vi "0 to 99 sub vi.vi"(1 "Numeric":dbl) -> (0 "String":string)   [LabVIEW 2020]
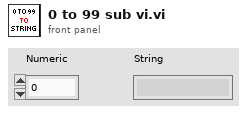
[diagram p1: front panel]
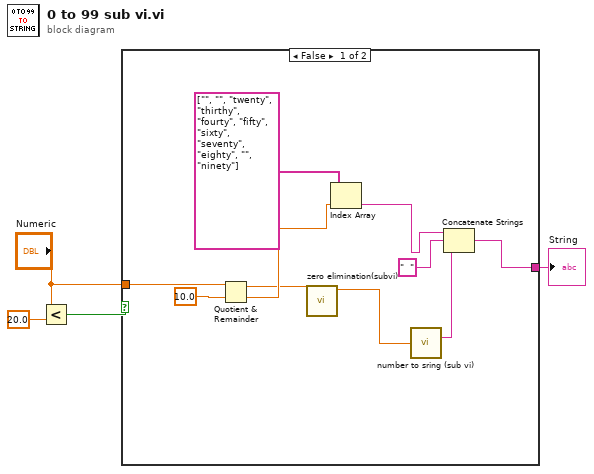
[diagram p0: block diagram]
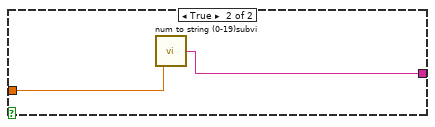
[diagram p2: hidden frame]
diagram:
  n1 = Less?(x="Numeric", y=20.0) -> (x < y?=w1:bool)
  n2 = case shown="False" w1 {
    tunnel: "Numeric" -> [w14 w16]
    tunnel: [w9 w15] -> w4
    frame False {
      n3 = Quotient & Remainder(x=w14, y=10.0) -> (x-y*floor(x/y)=w7:dbl, floor(x/y)=w8:dbl)
      n4 = call "zero elimination(subvi).vi"("Numeric"=w7) -> ("t"=w6:dbl)  [unwired: 10 in]
      n5 = Index Array(array=string[] ["", "", "twenty", "thirthy", "fourty", "fifty", "sixty", "seventy", "eighty", "", "ninety"], index=w8) -> (element=w11:string)
      n6 = call "number to sring (sub vi).vi"("Numeric"=w6) -> ("element"=w5:string)
      n7 = Concatenate Strings(w11, "  " ("string"), w5) -> (w9:string)
    }
    frame True {
      n8 = call "num to string (0-19)subvi.vi"("Numeric"=w16) -> ("element"=w15:string)
    }
  }
  "String" <- w4
